vi "Read Doc Hwnd.vi"(8 "error in (no error)":errorcluster, 11 "Document in":refnum<class "Document.lvclass">) -> (0 "error out":errorcluster, 2 "Child Hwnd":u32, 3 "Document out":refnum<class "Document.lvclass">)   [LabVIEW 2019, in "Document.lvclass"]
uses:
  Document.lvclass
  Document.lvclass/Document.ctl
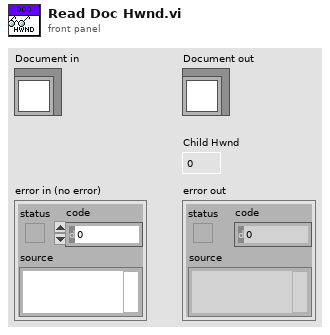
[diagram p1: front panel]
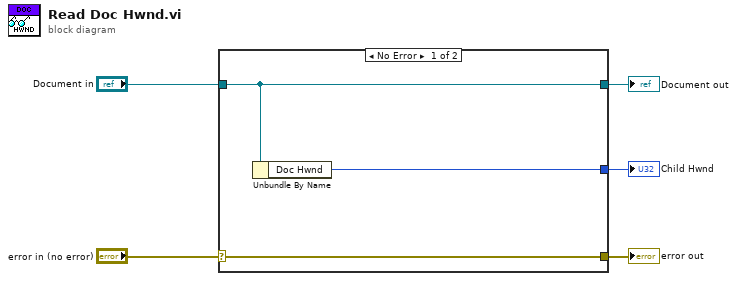
[diagram p0: block diagram]
diagram:
  n1 = case shown="No Error" "error in (no error)" {
    selector: "error in (no error)" -> [w8 w9]
    tunnel: [w8 w9] -> w4
    tunnel: [w7 w10] -> w2
    tunnel: "Document in" -> [w7 w10]
    tunnel: [w6 _] -> w1
    frame No Error {
      n2 = Unbundle By Name(w7) -> ("Doc Hwnd"=w6:u32)
    }
    frame Error {
    }
  }
  "error out" <- w4
  "Document out" <- w2
  "Child Hwnd" <- w1
